vi "Set Launcher Ping Response.vi"(7 "Streaming? (F)":bool, 8 "error in (no error)":errorcluster, 10 "Message Data":T1, 11 "gRPCid in":T5) -> (0 "error out":errorcluster)   [LabVIEW 2021, in "CIF_Launcher_server.lvlib" / "Launcher.lvclass"]
uses:
  Launcher.lvclass
  <vilib>/gRPC/LabVIEW gRPC Library/Shared/grpcId.ctl
  Launcher.lvclass/Launcher.ctl
  CIF_Launcher_server.lvlib
  <vilib>/gRPC/LabVIEW gRPC Library/grpc-lvsupport-release.lvlib
  RPC Messages/cif_common_Status.ctl
  RPC Messages/cif_manager_LauncherType.ctl
  RPC Messages/cif_manager_LauncherInfo.ctl
  RPC Messages/cif_manager_LauncherStatus.ctl
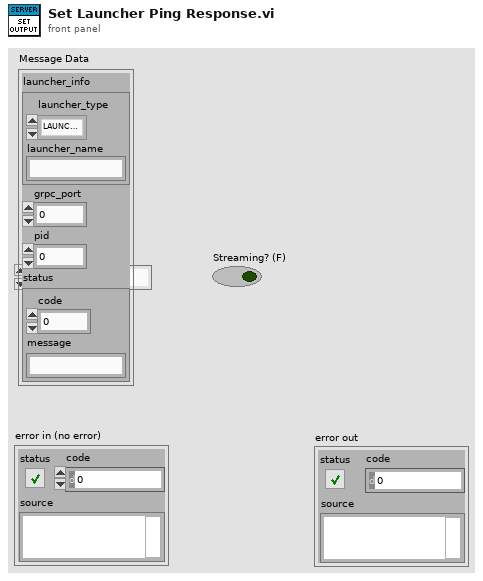
[diagram p1: front panel]
types:
  T1 = typedef "CIF_Launcher_server.lvlib/cif_manager_LauncherStatus.ctl" = cluster{"launcher_info":T2, "grpc_port":i32, "pid":u32, "status":T4}
  T2 = typedef "CIF_Launcher_server.lvlib/cif_manager_LauncherInfo.ctl" = cluster{"launcher_type":T3, "launcher_name":string}
  T3 = typedef "CIF_Launcher_server.lvlib/cif_manager_LauncherType.ctl" = enum32{"LAUNCHERTYPE_UNKNOWN", "LAUNCHERTYPE_LABVIEW"}
  T4 = typedef "CIF_Launcher_server.lvlib/cif_common_Status.ctl" = cluster{"code":i32, "message":string}
  T5 = typedef "grpc-lvsupport-release.lvlib/grpcId.ctl" = u64
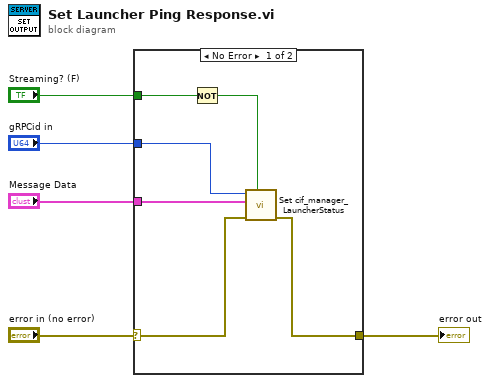
[diagram p0: block diagram]
diagram:
  n1 = case shown="No Error" "error in (no error)" {
    selector: "error in (no error)" -> [w11 w12]
    tunnel: [w9 w12] -> w4
    tunnel: "gRPCid in" -> [w10 _]
    tunnel: "Message Data" -> [w8 _]
    tunnel: "Streaming? (F)" -> [w7 _]
    frame No Error {
      n2 = Not(x=w7) -> (.not. x?=w6:bool)
      n3 = call "Set cif_manager_LauncherStatus.vi"("Complete Call (T)"=w6, "error in (no error)"=w11, "package_templatemessage"=w8, "gRPCid"=w10) -> ("error out"=w9:errorcluster)  [unwired: 7 in]
    }
    frame Error {
    }
  }
  "error out" <- w4
